vi "Get VI FQN.vi"(1 "Message":refnum<class "Async Message.lvclass">) -> (0 "String":string)   [LabVIEW 2023, in "Async Methods Actor.lvlib" / "Async Methods Actor.lvclass"]
uses:
  Async Methods Actor.lvclass
  Async Methods Actor Messages/Async Message/Async Message.lvclass
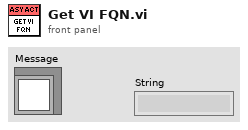
[diagram p1: front panel]
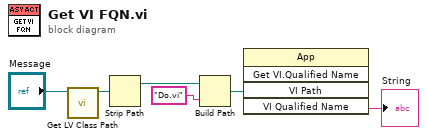
[diagram p0: block diagram]
diagram:
  n1 = call <vilib>:"Get LV Class Path.vi"("object"="Message") -> ("class path"=w5:path)  [unwired: 9 in, 1 out]
  n2 = Strip Path(path=w5) -> (stripped path=w4:path)  [unwired: 1 out]
  n3 = Build Path(base path=w4, name or relative path="Do.vi") -> (appended path=w1:path)
  n4 = invoke class="App" method="Get VI.Qualified Name"("VI Path"=w1) -> ("VI Qualified Name"=→"String":string)  [unwired: 4 in, 4 out]
